vi "init.vi"(8 "error in (no error)":errorcluster, 9 "Digital Signal Level":T1, 10 "DAQ Channel To Write":refnum<k21>, 11 "ConfigureILCDIStrategy in":refnum<class "ConfigureILCDIStrategy.lvclass">) -> (0 "error out":errorcluster, 3 "ConfigureILCDIStrategy out":refnum<class "ConfigureILCDIStrategy.lvclass">)   [LabVIEW 2015, in "ConfigureILCDIStrategy.lvclass"]
uses:
  ConfigureILCDIStrategy/ConfigureILCDIStrategy.lvclass
  Typedefs/Digital Signal Level.ctl
  ConfigureILCDIStrategy/ConfigureILCDIStrategy.lvclass/ConfigureILCDIStrategy.ctl
  Typedefs/ILCBTTypedefs.lvlib
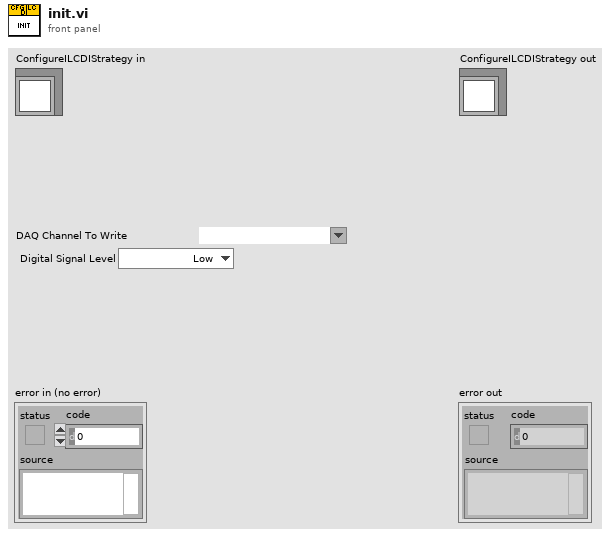
[diagram p1: front panel]
types:
  T1 = typedef "ILCBTTypedefs.lvlib/Digital Signal Level.ctl" = enum16{"Low", "High"}
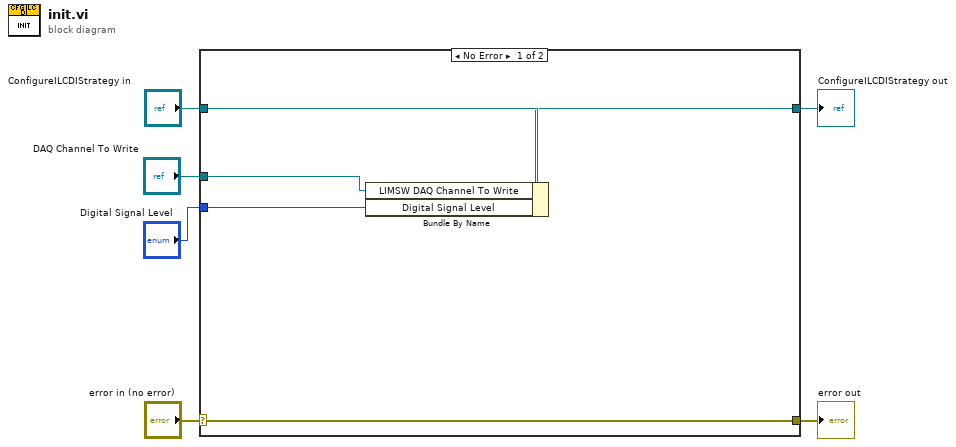
[diagram p0: block diagram]
diagram:
  n1 = case shown="No Error" "error in (no error)" {
    selector: "error in (no error)" -> [w11 w13]
    tunnel: [w11 w13] -> w5
    tunnel: [w9 w12] -> w3
    tunnel: "ConfigureILCDIStrategy in" -> [w10 w12]
    tunnel: "Digital Signal Level" -> [w8 _]
    tunnel: "DAQ Channel To Write" -> [w7 _]
    frame No Error {
      n2 = Bundle By Name(cluster=w10, "LIMSW DAQ Channel To Write"=w7, "Digital Signal Level"=w8) -> (w9:refnum<class "ConfigureILCDIStrategy.lvclass">)
    }
    frame Error {
    }
  }
  "error out" <- w5
  "ConfigureILCDIStrategy out" <- w3
